vi "Load.vi"(8 "error in (no error)":errorcluster, 10 "Exclusion Groups":string[](array[string]), 11 "TDMS File Path":path) -> (0 "error out":errorcluster, 1 "Success?":bool, 3 "TDMS File.":refnum<class "File.lvclass">)   [LabVIEW 2020, in "TDMS.lvlib"]
doc: "Load all data (except Data from the 'Exclusion Groups') from the TDMS file at 'TDMS File Path'. The data is stored on the TDMS File class."
uses:
  TDMS.lvlib
  TDMS File/File.lvclass
  TDMS Group/Group.lvclass/Group.ctl
  TDMS File/File.lvclass/File.ctl
  PPL/HDH.Data.Generic.lvlibp/Utility/Wrap In Generic.vi
  PPL/HDH.Data.Generic.lvlibp/Generic Data/Variant/Set Attribute.vi
  PPL/HDH.Data.Generic.lvlibp/Generic Data/Variant/Variant.lvclass
  TDMS Group/Group.lvclass
  TDMS Channel/Channel.lvclass
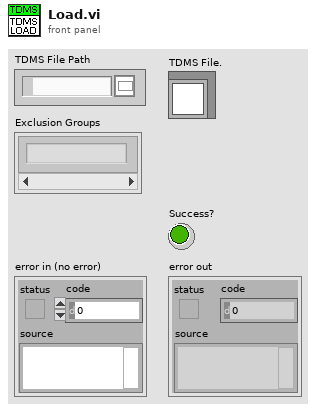
[diagram p1: front panel]
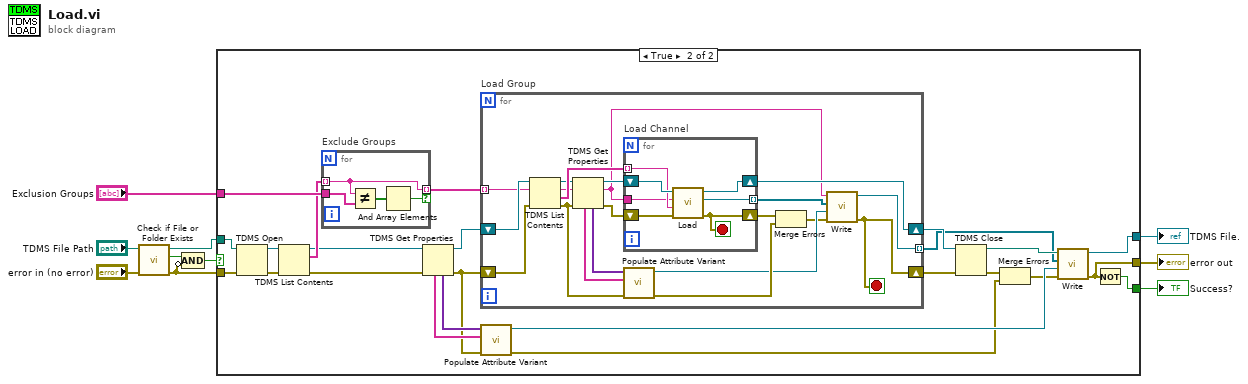
[diagram p0: block diagram]
diagram:
  n1 = call <vilib>:"Check if File or Folder Exists.vi"("error in (no error)"="error in (no error)", "path"="TDMS File Path") -> ("error out"=w7:errorcluster, "file or folder exists?"=w9:bool, "dup path"=w5:path)  [unwired: 7 in]
  n2 = Compound Arithmetic op=AND(w9, invert w7) -> (w6:bool)
  n3 = case shown="True" w6 {
    selector: w6 -> [w11 _]
    tunnel: [w12 w14] -> w2
    tunnel: w7 -> [w12 w35]
    tunnel: w5 -> [_ w36]
    tunnel: "Exclusion Groups" -> [_ w30]
    tunnel: [_ w15] -> w3
    tunnel: [w11 w13] -> w1
    frame False {
    }
    frame True {
      n4 = TDMS Open(8:w35, 11:w36) -> (0:w33:errorcluster, 3:w34:refnum<k34>)  [unwired: 5 in]
      n5 = TDMS List Contents(4:w33, 7:w34) -> (0:w25:errorcluster, 2:w29:string[], 3:w27:refnum<k34>)  [unwired: 1 in, 1 out]
      n6 = for "Exclude Groups" {
        tunnel: w30 -> [w40]
        tunnel: w29 -> [w39] mode=indexing
        tunnel: [w39] -> w28 mode=indexing if=w37
        n7 = Not Equal?(x=w39, y=w40) -> (x != y?=w38:bool[])
        n8 = And Array Elements(Boolean array=w38) -> (logical AND=w37:bool)
      }
      n9 = TDMS Get Properties(8:w25, 11:w27) -> (0:w22:errorcluster, 3:w26:refnum<k34>, 4:w24:variant[], 6:w23:string[])  [unwired: 4 in, 2 out]
      n10 = for "Load Group" {
        shift-right: [w57] -> w32
        shift-left: w26 -> [w60]
        tunnel: w28 -> [w51] mode=indexing
        shift-right: [w41] -> w31
        shift-left: w22 -> [w59]
        tunnel: [w42] -> w20 mode=indexing
        stop <- w41 stop-if-true
        n11 = TDMS List Contents(4:w59, 6:w51, 7:w60) -> (0:w50:errorcluster, 1:w58:string[], 2:w47:string, 3:w56:refnum<k34>)
        n12 = TDMS Get Properties(8:w50, 10:w47, 11:w56) -> (0:w54:errorcluster, 2:w46:string, 3:w55:refnum<k34>, 4:w53:variant[], 6:w52:string[])  [unwired: 3 in, 1 out]
        n13 = for "Load Channel" {
          tunnel: w58 -> [w65] mode=indexing
          shift-right: [w62] -> w57
          shift-left: w55 -> [w67]
          shift-right: [w64] -> w48
          shift-left: w54 -> [w66]
          tunnel: w46 -> [w63]
          tunnel: [w61] -> w44 mode=indexing
          stop <- w64 stop-if-true
          n14 = call "Load.vi"("error in (no error)"=w66, "Channel Name"=w65, "Group Name"=w63, "tdms file in"=w67) -> ("error out"=w64:errorcluster, "Channel out"=w61:refnum<class "Channel.lvclass">, "tdms file out"=w62:refnum<k34>)  [unwired: 5 in]
        }
        n15 = call "Populate Attribute Variant.vi"("error in (no error)"=w50, "Property Names"=w52, "Property Values"=w53) -> ("error out"=w49:errorcluster, "Attribute Variant out"=w45:refnum<class "Variant.lvclass">)  [unwired: 7 in]
        n16 = Merge Errors(w48, w49) -> (w43:errorcluster)
        n17 = call "Write.vi"("error in (no error)"=w43, "Group Properties"=w45, "Channels"=w44, "Group Name"=w46) -> ("error out"=w41:errorcluster, "TDMS Group out"=w42:refnum<class "Group.lvclass">)  [unwired: 6 in]
      }
      n18 = call "Populate Attribute Variant.vi"("error in (no error)"=w22, "Property Names"=w23, "Property Values"=w24) -> ("error out"=w17:errorcluster, "Attribute Variant out"=w19:refnum<class "Variant.lvclass">)  [unwired: 7 in]
      n19 = TDMS Close(8:w31, 11:w32) -> (0:w18:errorcluster, 3:w21:path)
      n20 = Merge Errors(w18, w17) -> (w16:errorcluster)
      n21 = call "Write.vi"("error in (no error)"=w16, "File Properties"=w19, "Groups"=w20, "File Path"=w21) -> ("error out"=w14:errorcluster, "TDMS File out"=w15:refnum<class "File.lvclass">)  [unwired: 6 in]
      n22 = Not(x=w14) -> (.not. x?=w13:bool)
    }
  }
  "error out" <- w2
  "TDMS File." <- w3
  "Success?" <- w1
